vi "README example get.vi"() -> ()   [LabVIEW 2013]
uses:
  infolib.lvlib
  Private/Get key polymorph parts/GetEXT.vi
  Private/Get key polymorph parts/GetString.vi
  Private/Get key polymorph parts/GetTime Stamp.vi
panel:
  out "forg_codes":string
  out "start":timestamp
  out "all_codes":string
  out "chars":string
  out "colour":string
  out "length":ext format="%#_20g"
  in  "info data in":string="Measured length (mm):: 34.123456789000000000\r\nColour of my car:: gold metallic\r\nrAnDoM CHarACteRS:: @#$%^&()43]}øèe\r\n#startsection:: known codes\r\n        IDDQD\n        IDKFA\n\r        #startsection:: forgotten codes\r\n                IDSPISPOPD\n                IDBEHOLDL\n                IDBEHOLDR\r\n        #endsection:: forgotten codes\n#endsection:: known codes\r\nNote: the above codes are not valid for most\nof devices in the local reality.\r\n#startmatrix:: list of my favorite numbers\r\n        1.0000000000000000000; 11.000000000000000000; 42.000000000000000000; \r\n        3333.0000000000000000; 999999999999999949000000000000000000000000000000000000000000000000000000; 0.0000000000000000000; \r\n        -1.0000000000000000000; -3333.0000000000000000; 0.0000010000000000000000000; \r\n#endmatrix:: list of my favorite numbers\r\nStart of measurement:: 2017-07-02T17:59:17.01978799999999999997\r"
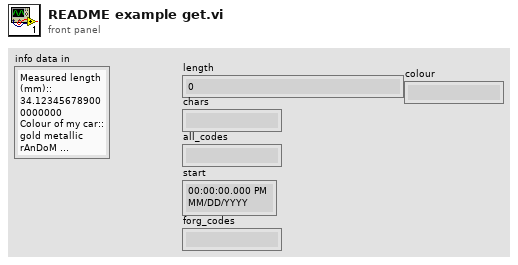
[diagram p1: front panel]
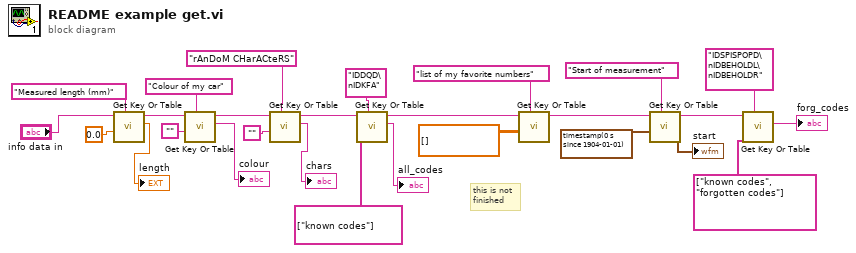
[diagram p0: block diagram]
diagram:
  # "this is not\nfinished"
  n1 = call-poly "Get Key Or Table.vi"("key description"="Measured length (mm)", "numeric"=0.0, "info data"="info data in") -> ("value"=→"length":ext, "info data out"=w23:string)  [unwired: 6 in, 1 out]
  n2 = call-poly "Get Key Or Table.vi"("key description"="Colour of my car", "string"="", "info data"=w23) -> ("value"=→"colour":string, "info data out"=w20:string)  [unwired: 6 in, 1 out]
  n3 = call-poly "Get Key Or Table.vi"("key description"="rAnDoM CHarACteRS", "string"="", "info data"=w20) -> ("value"=→"chars":string, "info data out"=w16:string)  [unwired: 6 in, 1 out]
  n4 = call-poly "Get Key Or Table.vi"("key description"="IDDQD\nIDKFA", "sections"=string[] ["known codes"], "info data"=w16) -> ("value"=→"all_codes":string, "info data out"=w14:string)  [unwired: 6 in, 1 out]
  n5 = call-poly "Get Key Or Table.vi"("key description"="list of my favorite numbers", "numeric"=ext[][] [], "info data"=w14) -> ("info data out"=w13:string)  [unwired: 6 in, 2 out]
  n6 = call-poly "Get Key Or Table.vi"("key description"="Start of measurement", "time stamp"=timestamp(0 s since 1904-01-01), "info data"=w13) -> ("value"=→"start":timestamp, "info data out"=w8:string)  [unwired: 6 in, 1 out]
  n7 = call-poly "Get Key Or Table.vi"("key description"="IDSPISPOPD\nIDBEHOLDL\nIDBEHOLDR" ("info data to insert"), "sections"=string[] ["known codes", "forgotten codes"], "info data"=w8) -> ("value"=→"forg_codes":string)  [unwired: 6 in, 2 out]
